vi "pmu_Close Time Queue.vi"(8 "error in (no error)":errorcluster, 11 "system info in":refnum<class "PMU System Info.lvclass">) -> (0 "error out":errorcluster)   [LabVIEW 2011, in "NI_EP_PMU.lvlib" / "PMU System Info.lvclass"]
uses:
  <vilib>/addons/Electrical Power/PMU/Common/Classes/PMU System Info/PMU System Info.lvclass
  <vilib>/addons/Electrical Power/PMU/Common/Classes/PMU System Info/PMU System Info.lvclass/PMU System Info.ctl
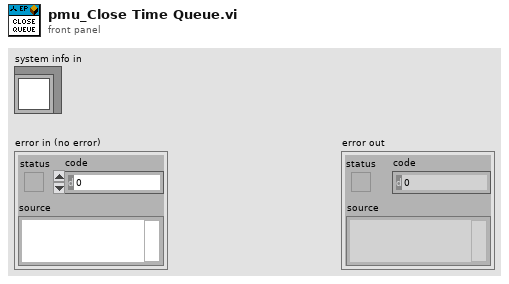
[diagram p1: front panel]
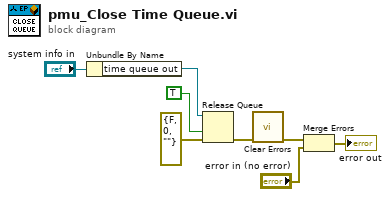
[diagram p0: block diagram]
diagram:
  n1 = Unbundle By Name("system info in") -> ("time queue out"=w5:refnum<queue>)
  n2 = Release Queue(queue=w5, force destroy? (F)=TRUE, error in (no error)=errorcluster {"status"=FALSE, "code"=0, "source"=""}) -> (error out=w4:errorcluster)  [unwired: 2 out]
  n3 = call <vilib>:"Clear Errors.vi"("error in (no error)"=w4) -> ("error out"=w2:errorcluster)  [unwired: 6 in]
  n4 = Merge Errors(w2, "error in (no error)") -> (→"error out":errorcluster)
